vi "Data Receiver_subvi.vi"(2 "stop flag":bool, 3 "error in":errorcluster, 4 "tdms file":refnum<k34>) -> (0 "warning out":errorcluster, 1 "tdmserror out":errorcluster)   [LabVIEW 2024]
doc: "Demonstrates how to open a connection to a specified host and port, read the data being sent to the port, and display the data on a chart. This VI is designed to stop if the TCP connection is terminated.\n\n<B>Note:</B> Requires the Simple Data Server.vi located in the same library as this VI."
panel:
  out "Time":string
  out "Bytes to read (dec)":i32
  out "Bytes to read (hex)":string
  out "Complete String after 'Bytes to read'":string
  out "Peak Powers":string[][](array[string])
  out "Peak Wavelengths":string[][](array[string])
  out "System Status":string[][](array[string])
  out "Qty of FBG's":string[](array[string])
  out "OpticalLineNumber":string[](array[string])
  out "Date":string
  out "LineNumber":string
  out "Qty of Optical Lines":string
  in  "Start":bool
  in  "Address":string="127.0.0.1"
  in  "Port":u16=2055 min=1025 step=1
  # "Instructions:\n1. Adjust the IP address and Port.\n2. Press START."
  # "Separated data"
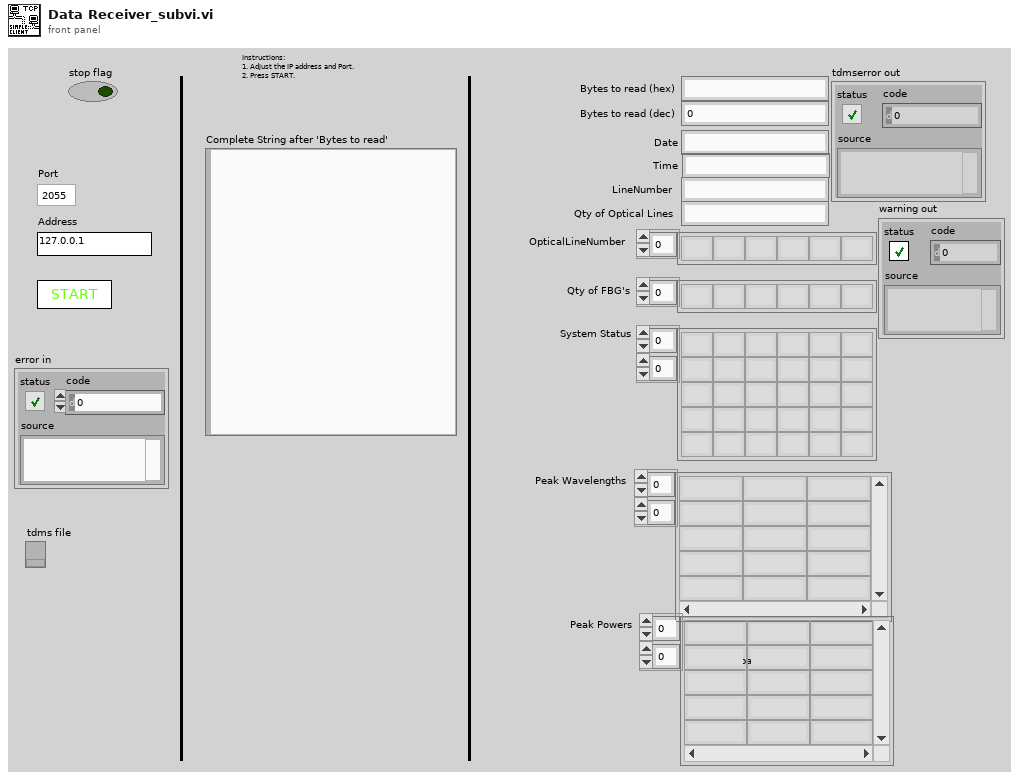
[diagram p1: front panel]
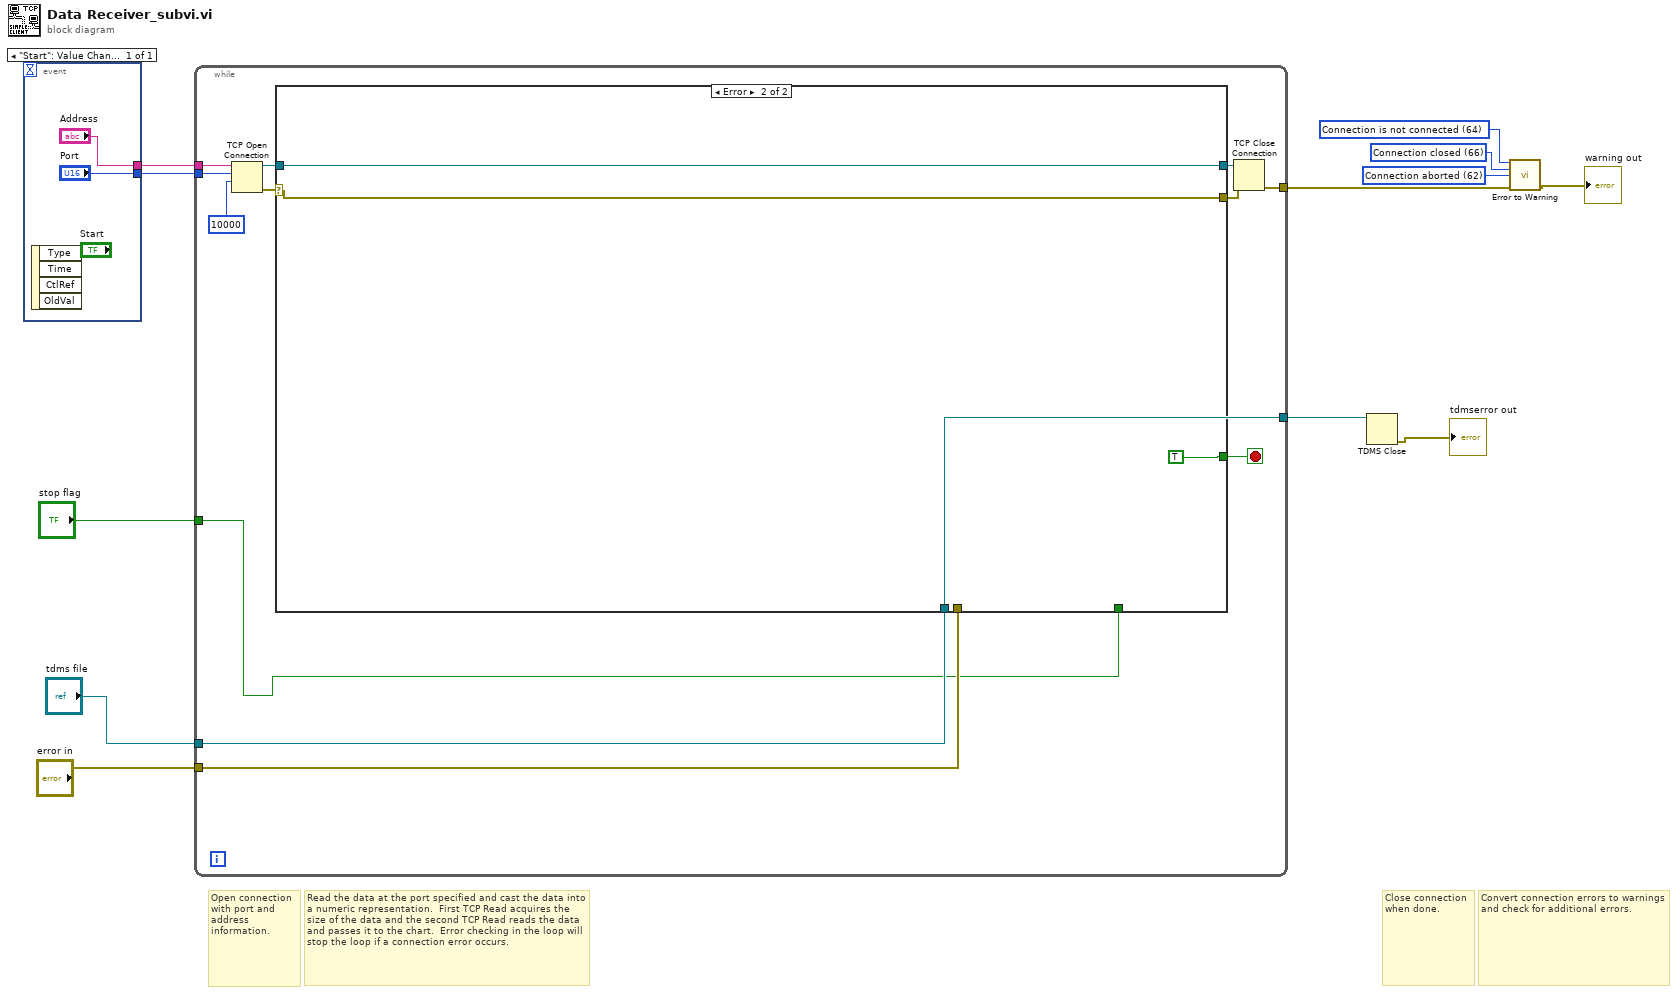
[diagram p0: block diagram]
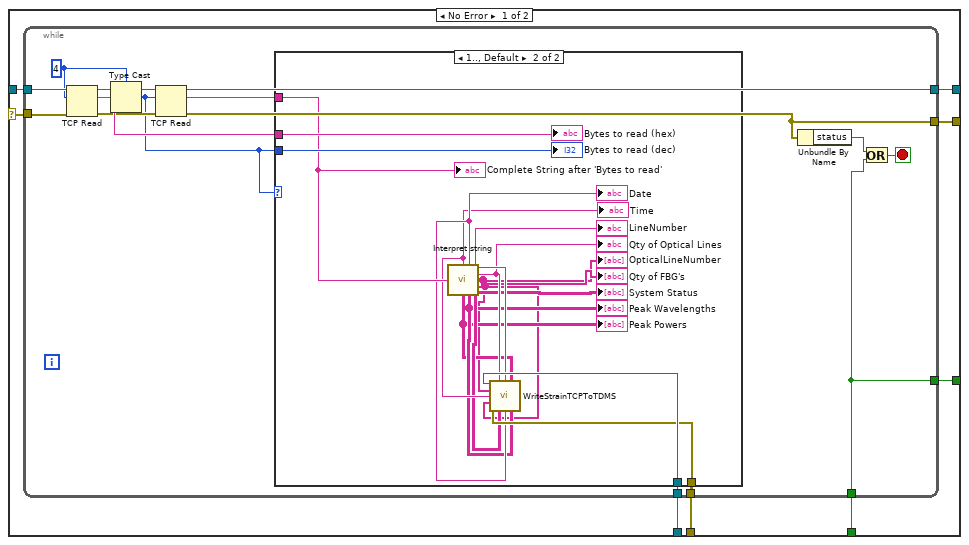
[diagram p2: hidden frame]
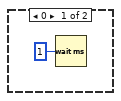
[diagram p3: hidden frame]
diagram:
  w9 = 62 items=["No Error", "Argument Error", "Memory Full", "Out of Zone", "End of File", "File Already Open", "Generic File IO Error", "File Not Found", "File Permission Error", "Disk Full", "Duplicate Path", "Too Many Files Open", "Not Enabled", "Resource File Not Found", "Cannot Add Resource", "Resource Not Found", "Image Not Found", "Image Memory Error", "Pen Does Not Exist", "Config Bad Type", "Config Token Not Found", "Config Parse Error", "Config Memory Error", "Bad External Code Format", "Bad External Code Offset", "External Code Not Present", "Null Window", "Destroy Window Mixup", "Null Menu", "Print Aborted", "Bad Print Record", "Print Driver Error", "Windows Error During Print", "Memory Error During Print", "Print Dialog Error", "Generic Print Error", "Invalid Device Refnum", "Device Not Found", "Device Parameter Error", "Device Unit Error", "Can't Open Device", "Device Call Aborted", "Generic Error", "Cancelled By User", "Object ID Too Low", "Object ID Too High", "Object Not In Heap", "Unknown Heap", "Bad DefProc ID", "DefProc Not In Table", "Message Out Of Range", "Null Method", "Unknown Message", "Manager Call Not Supported", "Bad address", "Connection In progress", "Connection timed out", "Connection is already in progress", "Network attribute not supported", "Network error", "Address in use", "System out of memory", "Connection aborted", "Connection refused", "Connection is not connected", "Connection is already connected", "Connection closed", "Initialize error (interapplication manager)", "Bad occurrence", "Wait on unbound occurrence handler", "Occurrence queue overflow", "Bad path", "Semaphore not signaled", "Unrecognized type (interapplication manager)"] ("1st Error to Convert")
  w10 = 66 items=["No Error", "Argument Error", "Memory Full", "Out of Zone", "End of File", "File Already Open", "Generic File IO Error", "File Not Found", "File Permission Error", "Disk Full", "Duplicate Path", "Too Many Files Open", "Not Enabled", "Resource File Not Found", "Cannot Add Resource", "Resource Not Found", "Image Not Found", "Image Memory Error", "Pen Does Not Exist", "Config Bad Type", "Config Token Not Found", "Config Parse Error", "Config Memory Error", "Bad External Code Format", "Bad External Code Offset", "External Code Not Present", "Null Window", "Destroy Window Mixup", "Null Menu", "Print Aborted", "Bad Print Record", "Print Driver Error", "Windows Error During Print", "Memory Error During Print", "Print Dialog Error", "Generic Print Error", "Invalid Device Refnum", "Device Not Found", "Device Parameter Error", "Device Unit Error", "Can't Open Device", "Device Call Aborted", "Generic Error", "Cancelled By User", "Object ID Too Low", "Object ID Too High", "Object Not In Heap", "Unknown Heap", "Bad DefProc ID", "DefProc Not In Table", "Message Out Of Range", "Null Method", "Unknown Message", "Manager Call Not Supported", "Bad address", "Connection In progress", "Connection timed out", "Connection is already in progress", "Network attribute not supported", "Network error", "Address in use", "System out of memory", "Connection aborted", "Connection refused", "Connection is not connected", "Connection is already connected", "Connection closed", "Initialize error (interapplication manager)", "Bad occurrence", "Wait on unbound occurrence handler", "Occurrence queue overflow", "Bad path", "Semaphore not signaled", "Unrecognized type (interapplication manager)"] ("1st Error to Convert")
  w11 = 64 items=["No Error", "Argument Error", "Memory Full", "Out of Zone", "End of File", "File Already Open", "Generic File IO Error", "File Not Found", "File Permission Error", "Disk Full", "Duplicate Path", "Too Many Files Open", "Not Enabled", "Resource File Not Found", "Cannot Add Resource", "Resource Not Found", "Image Not Found", "Image Memory Error", "Pen Does Not Exist", "Config Bad Type", "Config Token Not Found", "Config Parse Error", "Config Memory Error", "Bad External Code Format", "Bad External Code Offset", "External Code Not Present", "Null Window", "Destroy Window Mixup", "Null Menu", "Print Aborted", "Bad Print Record", "Print Driver Error", "Windows Error During Print", "Memory Error During Print", "Print Dialog Error", "Generic Print Error", "Invalid Device Refnum", "Device Not Found", "Device Parameter Error", "Device Unit Error", "Can't Open Device", "Device Call Aborted", "Generic Error", "Cancelled By User", "Object ID Too Low", "Object ID Too High", "Object Not In Heap", "Unknown Heap", "Bad DefProc ID", "DefProc Not In Table", "Message Out Of Range", "Null Method", "Unknown Message", "Manager Call Not Supported", "Bad address", "Connection In progress", "Connection timed out", "Connection is already in progress", "Network attribute not supported", "Network error", "Address in use", "System out of memory", "Connection aborted", "Connection refused", "Connection is not connected", "Connection is already connected", "Connection closed", "Initialize error (interapplication manager)", "Bad occurrence", "Wait on unbound occurrence handler", "Occurrence queue overflow", "Bad path", "Semaphore not signaled", "Unrecognized type (interapplication manager)"] ("1st Error to Convert")
  # "Convert connection errors to warnings and check for additional errors."
  # "Close connection when done."
  # "Read the data at the port specified and cast the data into a numeric representation.  First TCP Read acquires the size of the data and the second TCP Read reads the data and passes it to the chart.  Error checking in the loop will stop the loop if a connection error occurs."
  # "Open connection\nwith port and \naddress information."
  n1 = event shown="[0] \"Start\": Value Change" {
    selector: _ -> [_]
    dyn-events: _ -> [_]
    timeout: _ -> [_]
    tunnel: ["Address"] -> w8
    tunnel: ["Port"] -> w7
    event "Start": Value Change {
      n2 = event-data() -> ()  [unwired: 1 in, 4 out]
    }
  }
  n3 = while {
    tunnel: [w23] -> w12
    tunnel: w8 -> [w22]
    tunnel: w7 -> [w21]
    tunnel: "tdms file" -> [w16]
    tunnel: "error in" -> [w17]
    tunnel: [w16] -> w6
    tunnel: "stop flag" -> [w15]
    stop <- w20 stop-if-true
    n4 = TCP Open Connection(address=w22, remote port or service name=w21, timeout ms (60000)=10000) -> (connection ID=w24:refnum<k5>, error out=w19:errorcluster)  [unwired: 2 in]
    n5 = case shown="Error" w19 {
      selector: w19 -> [w30 w66]
      tunnel: [w34 w66] -> w26
      tunnel: [w33 w67] -> w25
      tunnel: w24 -> [w32 w67]
      tunnel: [w31 TRUE] -> w20
      tunnel: w16 -> [w29 _]
      tunnel: w17 -> [w28 _]
      tunnel: w15 -> [w27 _]
      frame No Error {
        n6 = while {
          tunnel: w30 -> [w46]
          tunnel: w32 -> [w47]
          tunnel: [w48] -> w33
          tunnel: [w45] -> w34
          tunnel: [w35] -> w31
          tunnel: w29 -> [w37]
          tunnel: w28 -> [w36]
          tunnel: w27 -> [w35]
          stop <- w43 stop-if-true
          w39 = 4
          n7 = TCP Read(connection ID=w47, bytes to read=w39, error in (no error)=w46) -> (connection ID out=w49:refnum<k5>, data out=w42:string, error out=w40:errorcluster)  [unwired: 2 in]
          n8 = Type Cast(type=w39, x=w42) -> (*(type *) &x=w38:i32)
          n9 = TCP Read(connection ID=w49, bytes to read=w38, error in (no error)=w40) -> (connection ID out=w48:refnum<k5>, data out=w41:string, error out=w45:errorcluster)  [unwired: 2 in]
          n10 = case shown="1.., Default" w38 {
            tunnel: w42 -> [_ w64]
            tunnel: w41 -> [_ w62]
            tunnel: w38 -> [_ w63]
            tunnel: w37 -> [_ w61]
            tunnel: w36 -> [_ w60]
            frame 0 {
              n11 = Wait (ms)(milliseconds to wait=u32 1) -> ()  [unwired: 1 out]
            }
            frame 1.., Default {
              n12 = call "Interpret string.vi"("Spreadsheet string"=w62) -> ("Time"=w58:string, "Date"=w59:string, "LineNumber"=w57:string, "Qty of Optical Lines"=w56:string, "OpticalLineNumber"=w51:string[], "Qty of FBG's"=w52:string[], "Peak Powers"=w53:string[][], "Peak Wavelengths"=w54:string[][], "System Status"=w55:string[][])  [unwired: 6 in]
              "Qty of Optical Lines" <- w56
              "LineNumber" <- w57
              "Date" <- w59
              "OpticalLineNumber" <- w51
              "Qty of FBG's" <- w52
              "System Status" <- w55
              "Peak Wavelengths" <- w54
              "Peak Powers" <- w53
              "Time" <- w58
              n13 = call "WriteStrainTCPToTDMS.vi"("Refnum in"=w61, "Qty of Optical Lines"=w56, "LineNumber"=w57, "Peak Powers"=w53, "OpticalLineNumber"=w51, "Time"=w58, "Qty of FBG's"=w52, "error in (no error)"=w60, "System Status"=w55, "Date"=w59, "Peak Wavelengths"=w54) -> ()  [unwired: 5 in]
              "Complete String after 'Bytes to read'" <- w62
              "Bytes to read (hex)" <- w64
              "Bytes to read (dec)" <- w63
            }
          }
          n14 = Unbundle By Name(w45) -> ("status"=w44:bool)
          n15 = Or(x=w44, y=w35) -> (x .or. y?=w43:bool)
        }
      }
      frame Error {
      }
    }
    n16 = TCP Close Connection(connection ID=w25, error in (no error)=w26) -> (error out=w23:errorcluster)  [unwired: 1 in, 1 out]
  }
  n17 = TDMS Close(11:w6) -> (0:→"tdmserror out":errorcluster)  [unwired: 1 in, 1 out]
  n18 = call <vilib>:"Error to Warning.vi"("1st Error to Convert"=w11, "2nd Error to Convert"=w10, "3rd Error to Convert"=w9, "error in"=w12) -> ("warning out"=→"warning out":errorcluster)  [unwired: 11 in]
